vi "Tosca-2P-Show Start Message.vi"() -> ()   [LabVIEW 2020]
panel:
  out "Message":string
  in  "Continue Button":bool
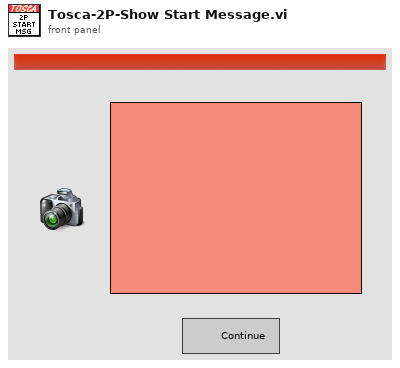
[diagram p1: front panel]
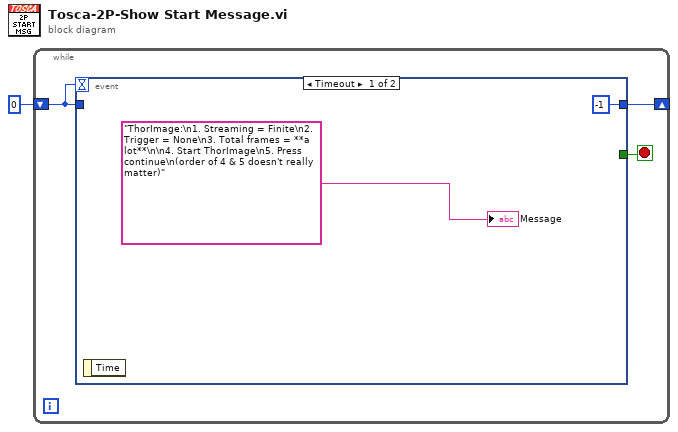
[diagram p0: block diagram]
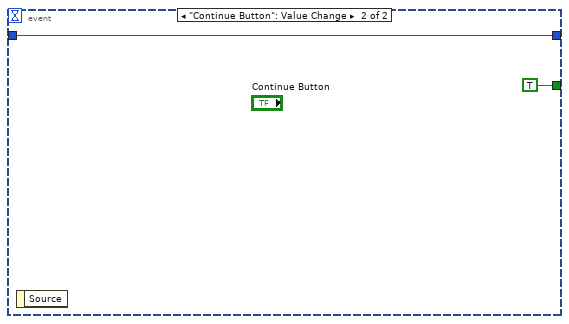
[diagram p2: hidden frame]
diagram:
  n1 = while {
    shift-right: [w3] -> _
    shift-left: 0 -> [w4]
    stop <- w2 stop-if-true
    n2 = event shown="[0] Timeout" {
      selector: _ -> [_ _]
      dyn-events: _ -> [_ _]
      timeout: w4 -> [_ _]
      tunnel: w4 -> [_ w8]
      tunnel: [-1 w8] -> w3
      tunnel: [_ TRUE] -> w2
      event Timeout {
        n3 = event-data() -> ()  [unwired: 1 in, 1 out]
        "Message" <- "ThorImage:\n1. Streaming = Finite\n2. Trigger = None\n3. Total frames = **a lot**\n\n4. Start ThorImage\n5. Press continue\n(order of 4 & 5 doesn't really matter)" ("Message 2")
      }
      event "Continue Button": Value Change {
        n4 = event-data() -> ()  [unwired: 1 in, 1 out]
      }
    }
  }
